vi "sendValue.vi"(8 "error in (no error)":errorcluster, 10 "data":variant, 11 "dropoutDoorState in":refnum<class "dropoutDoorState.lvclass">) -> (0 "error out":errorcluster, 2 "function return":i32, 3 "dropoutDoorState out":refnum<class "dropoutDoorState.lvclass">)   [LabVIEW 2016, in "SALLV_AtDome_Messaging.lvlib" / "dropoutDoorState.lvclass"]
uses:
  dropoutDoorState.lvclass
  ts_sallv_AtDome/DataTypes/logevent_dropoutDoorState.ctl
  ts_sallv_AtDome/SALLV_AtDome.lvlib
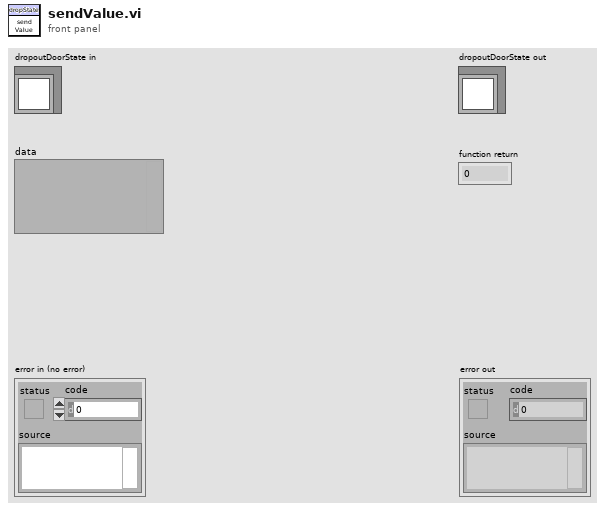
[diagram p1: front panel]
types:
  T1 = typedef "SALLV_AtDome.lvlib/logevent_dropoutDoorState.ctl" = cluster{"state":i32, "priority":i32}
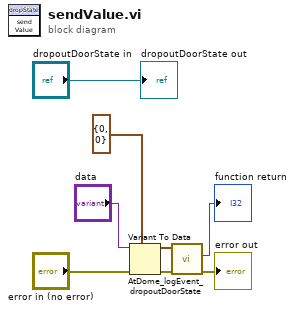
[diagram p0: block diagram]
diagram:
  n1 = Variant To Data(error in="error in (no error)", type=T1 {"state"=0, "priority"=0} ("logevent_dropoutDoorState_Ctl"), Variant="data") -> (data=w4:T1, error out=w5:errorcluster)
  n2 = call "AtDome_logEvent_dropoutDoorState.vi"("error in (no error)"=w5, "logevent_dropoutDoorState_Ctl"=w4) -> ("error out"=→"error out":errorcluster, "function return"=→"function return":i32)  [unwired: 7 in, 1 out]
  "dropoutDoorState out" <- "dropoutDoorState in"
